vi "LIA Digital PLL FPGA.vi"(5 "configuration":T1, 6 "arm":bool, 7 "reset":bool, 8 "m":i8, 9 "input valid":bool, 10 "q":fxp<+/-,48,0>, 11 "I":fxp<+/-,18,1>) -> (0 "value":i64, 1 "output valid":bool, 2 "accumulator":fxp<+/-,48,0>, 3 "frequency shift":fxp<+/-,48,0>)   [LabVIEW 2017]
uses:
  <instrlib>/_niInstr/Data Trigger/v1/Shared/Public/Edge Configuration FXP(+-,18,1).ctl
  <instrlib>/_niInstr/Data Trigger/v1/Shared/Public/Edge Configuration Trigger Slope.ctl
  <instrlib>/_niInstr/Data Trigger/v1/FPGA/Private/Trigger/Edge FXP(+-,18,1)x1spc.vi
  <instrlib>/_niInstr/Data Trigger/v1/FPGA/niInstr Data Trigger v1 FPGA.lvlib
  <instrlib>/_niInstr/Data Trigger/v1/Shared/niInstr Data Trigger v1 Shared.lvlib
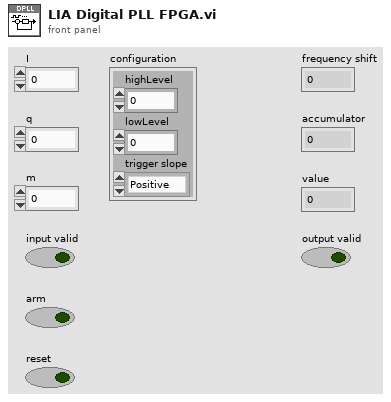
[diagram p1: front panel]
types:
  T1 = typedef "niInstr Data Trigger v1 Shared.lvlib/Edge Configuration FXP(+-,18,1).ctl" = cluster{"highLevel":fxp<+/-,18,1>, "lowLevel":fxp<+/-,18,1>, "trigger slope":T2}
  T2 = typedef "niInstr Data Trigger v1 Shared.lvlib/Edge Configuration Trigger Slope.ctl" = enum8{"Positive", "Negative"}
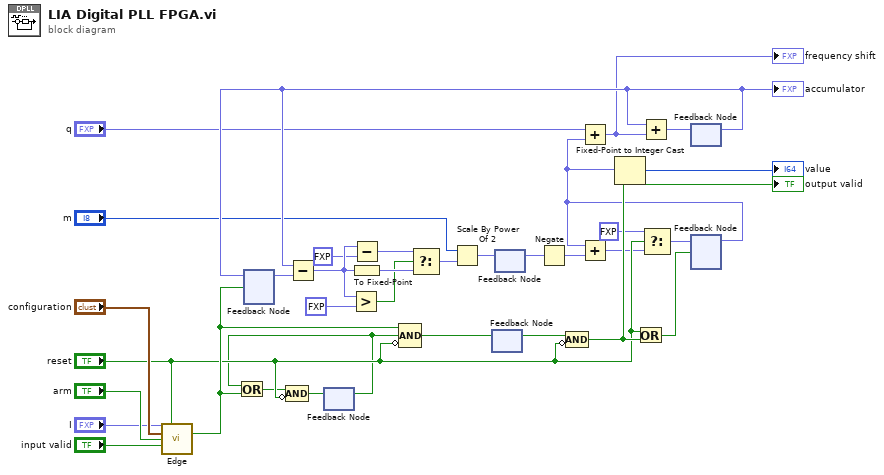
[diagram p0: block diagram]
diagram:
  n1 = call-poly <instrlib>:"Edge.vi"("data in"="I", "reset"="reset", "configuration"="configuration", "arm (T)"="arm", "input valid"="input valid") -> ("trigger"=w31:bool)  [unwired: 5 in, 5 out]
  n2 = feedback #1() -> (w2:fxp<+/-,48,0>)  [unwired: 1 in]
  n3 = feedback #2() -> (w18:bool)  [unwired: 1 in]
  n4 = Or(x=w18, y=w31) -> (x .or. y?=w16:bool)
  n5 = Compound Arithmetic op=AND(w16, invert "reset") -> (w17:bool)
  n6 = feedback-in #2(w17) -> ()
  n7 = Compound Arithmetic op=AND(w31, w18, invert "reset") -> (w20:bool)
  n8 = feedback #3() -> (w24:bool)  [unwired: 1 in]
  n9 = feedback-in #3(w20) -> ()
  n10 = feedback #4() -> (w23:fxp<+/-,48,0>)  [unwired: 1 in]
  n11 = Negate(x=w23) -> (-x=w10:fxp<+/-,48,0>)
  n12 = Compound Arithmetic op=AND(w24, invert "reset") -> (w34:bool)
  "output valid" <- w34
  n13 = Or(x="reset", y=w34) -> (x .or. y?=w15:bool)
  n14 = feedback #5() -> (w25:fxp<+/-,48,0>)  [unwired: 1 in]
  "accumulator" <- w25
  n15 = feedback-in #1(w25, w31) -> ()
  n16 = Subtract(x=w25, y=w2) -> (x-y=w11:fxp<+,48,0>)
  n17 = Greater?(x=w11, y=fxp<+,1,0> 0.5) -> (0:w4:bool)
  n18 = Subtract(x=w11, y=fxp<+,1,1> 1.0) -> (x-y=w6:fxp<+/-,48,0>)
  n19 = To Fixed-Point(number=w11) -> (fixed-point=w12:fxp<+/-,48,0>)  [unwired: 1 in]
  n20 = Select(t=w6, s=w4, f=w12) -> (s? t:f=w7:fxp<+/-,48,0>)
  n21 = Scale By Power Of 2(n="m", x=w7) -> (x*2^n=w8:fxp<+/-,48,0>)
  n22 = feedback-in #4(w8) -> ()
  n23 = feedback #6() -> (w32:fxp<+/-,48,0>)  [unwired: 1 in]
  n24 = Add(x="q", y=w32) -> (x+y=w22:fxp<+/-,48,0>)
  "frequency shift" <- w22
  n25 = Add(x=w32, y=w10) -> (x+y=w1:fxp<+/-,48,0>)
  n26 = Fixed-Point to Integer Cast(1:w32) -> (0:→"value":i64)
  n27 = Add(x=w25, y=w22) -> (x+y=w21:fxp<+/-,48,0>)
  n28 = Select(t=fxp<+/-,48,0> 0.0, s="reset", f=w1) -> (s? t:f=w19:fxp<+/-,48,0>)
  n29 = feedback-in #5(w21) -> ()
  n30 = feedback-in #6(w19, w15) -> ()
